vi "Read Headers_.vi"(8 "error in (no error)":errorcluster, 11 "CSV in":refnum<class "CSV.lvclass">) -> (0 "error out":errorcluster, 2 "Headers?":bool, 3 "CSV out":refnum<class "CSV.lvclass">)   [LabVIEW 2020, in "Manejador archivo.lvlib" / "CSV.lvclass"]
uses:
  CSV.lvclass
  CSV.lvclass/CSV.ctl
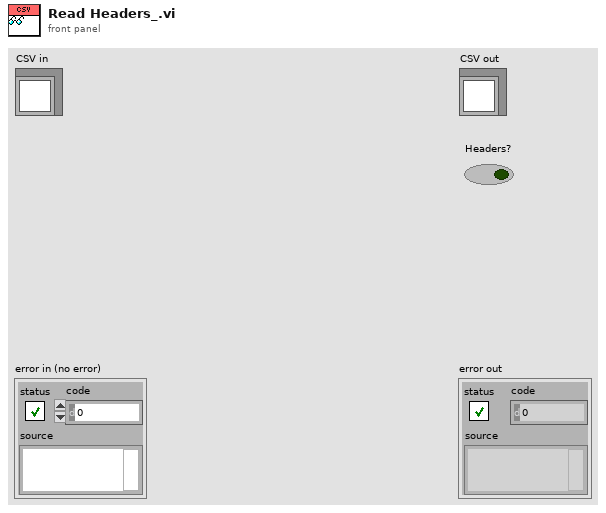
[diagram p1: front panel]
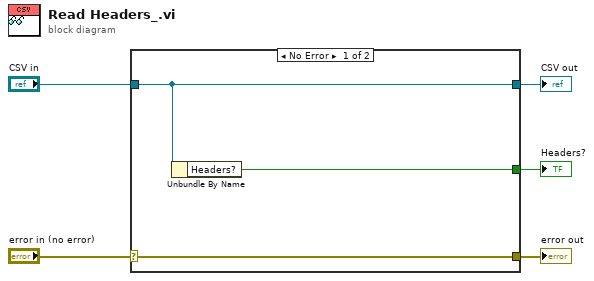
[diagram p0: block diagram]
diagram:
  n1 = case shown="No Error" "error in (no error)" {
    selector: "error in (no error)" -> [w8 w9]
    tunnel: [w8 w9] -> w4
    tunnel: [w7 w10] -> w2
    tunnel: "CSV in" -> [w7 w10]
    tunnel: [w6 _] -> w1
    frame No Error {
      n2 = Unbundle By Name(w7) -> ("Headers?"=w6:bool)
    }
    frame Error {
    }
  }
  "error out" <- w4
  "CSV out" <- w2
  "Headers?" <- w1
